vi "Parse Parameters.vi"(6 "error in (no error)":errorcluster, 9 "XML String In":string caption="Entrée de chaîne XML") -> (0 "error out":errorcluster, 3 "Params Values":T1(array[cluster]))   [LabVIEW 2022 SP3, in "EClib functions.lvlib"]
doc: "This intermediate VI transform a cluster of parameters to an array. This transformation is realised by XML Functions."
uses:
  EClib functions.lvlib
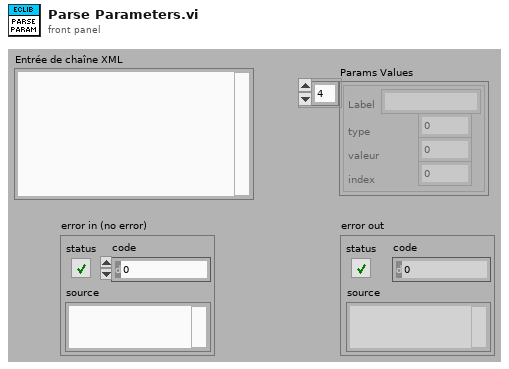
[diagram p1: front panel]
types:
  T1 = cluster{"Label":string, "type":i32, "valeur":u32, "index":i32}[]
  T2 = cluster{"string before end tag":string, i32, i32, i32}[]
  T3 = cluster{"string before end tag":string, i32, u32, i32}
  T4 = cluster{"string before end tag":string, i32, u32, i32}[]
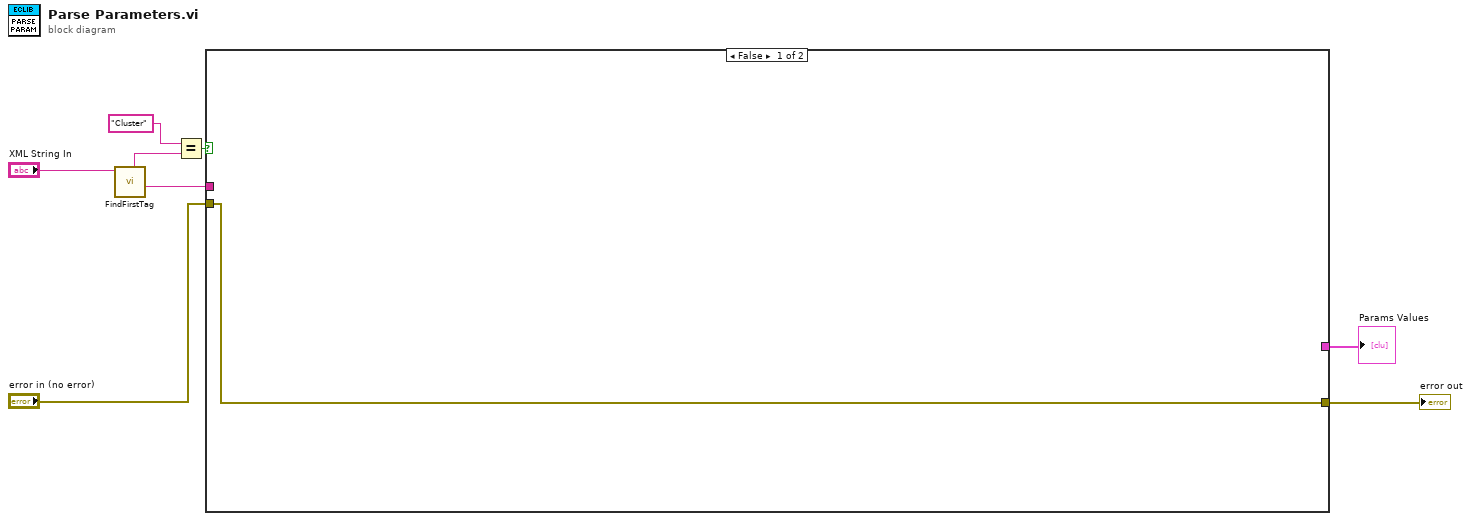
[diagram p0: block diagram]
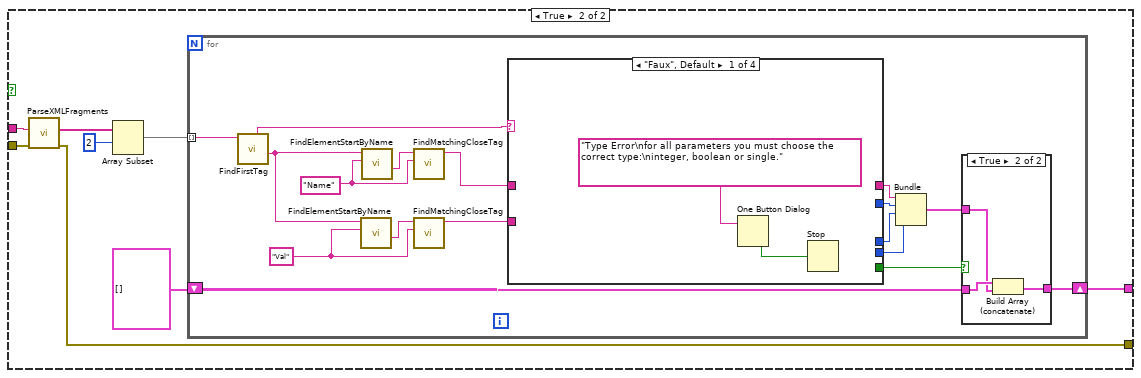
[diagram p2: hidden frame]
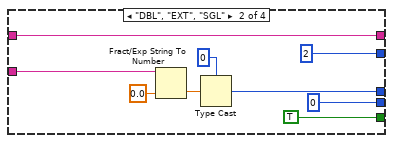
[diagram p4: hidden frame]
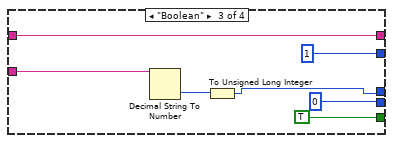
[diagram p5: hidden frame]
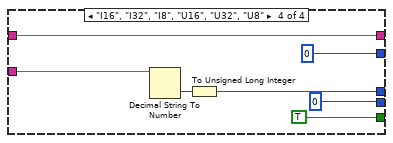
[diagram p6: hidden frame]
diagram:
  n1 = call <vilib>:"FindFirstTag.vi"("XML String In"="XML String In") -> ("after tag"=w7:string, "element name"=w3:string)  [unwired: 5 in, 4 out]
  n2 = Equal?(x="Cluster" ("y"), y=w3) -> (x = y?=w8:bool)
  n3 = case shown="False" w8 {
    tunnel: w7 -> [_ w17]
    tunnel: [_ w12] -> w6
    tunnel: "error in (no error)" -> [w9 w11]
    tunnel: [w9 w10] -> w1
    frame False {
    }
    frame True {
      n4 = call <vilib>:"ParseXMLFragments.vi"("error in (no error)"=w11, "XML in"=w17) -> ("error out"=w10:errorcluster, "XML Elements"=w16:string[])  [unwired: 8 in]
      n5 = Array Subset(array=w16, index=2 ("indice")) -> (w14:string[])  [unwired: 1 in]
      n6 = for {
        tunnel: w14 -> [w34] mode=indexing
        shift-right: [w26] -> w12
        shift-left: T2 [] -> [w28]
        w21 = "Val" ("Element Name")
        w25 = "Name" ("Element Name")
        n7 = call <vilib>:"FindFirstTag.vi"("XML String In"=w34) -> ("after tag"=w33:string, "element name"=w32:string)  [unwired: 5 in, 4 out]
        n8 = call <vilib>:"FindElementStartByName.vi"("Element Name"=w21, "string"=w33) -> ("after substring"=w22:string)  [unwired: 6 in, 3 out]
        n9 = call <vilib>:"FindElementStartByName.vi"("Element Name"=w25, "string"=w33) -> ("after substring"=w24:string)  [unwired: 6 in, 3 out]
        n10 = call <vilib>:"FindMatchingCloseTag.vi"("element name"=w25, "XML string in"=w24) -> ("string before end tag"=w23:string)  [unwired: 5 in, 4 out]
        n11 = call <vilib>:"FindMatchingCloseTag.vi"("element name"=w21, "XML string in"=w22) -> ("string before end tag"=w20:string)  [unwired: 5 in, 4 out]
        n12 = case shown="\"Faux\", Default" w32 {
          tunnel: w20 -> [_ w47 w53 w60]
          tunnel: w23 -> [_ w48 w55 w62]
          tunnel: [_ 2 1 0] -> w31
          tunnel: [_ w48 w55 w62] -> w19
          tunnel: [_ w43 w50 w57] -> w30
          tunnel: [_ TRUE TRUE TRUE] -> w29
          tunnel: [_ 0 0 0] -> w18
          frame "Faux", Default {
            n13 = One Button Dialog(message="Type Error\nfor all parameters you must choose the correct type:\ninteger, boolean or single.") -> (true=w39:bool)  [unwired: 1 in]
            n14 = Stop(stop? (T)=w39) -> ()
          }
          frame "DBL", "EXT", "SGL" {
            n15 = Fract/Exp String To Number(string=w47, default (0 dbl)=sgl 0.0 ("valeur par défaut (0 DBL)")) -> (number=w45:sgl)  [unwired: 2 in, 1 out]
            n16 = Type Cast(type=u32 0, x=w45) -> (*(type *) &x=w43:u32)
          }
          frame "Boolean" {
            n17 = Decimal String To Number(string=w53) -> (number=w51:i32)  [unwired: 2 in, 1 out]
            n18 = To Unsigned Long Integer(number=w51) -> (unsigned 32bit integer=w50:u32)
          }
          frame "I16", "I32", "I8", "U16", "U32", "U8" {
            n19 = Decimal String To Number(string=w60) -> (number=w59:i32)  [unwired: 2 in, 1 out]
            n20 = To Unsigned Long Integer(number=w59) -> (unsigned 32bit integer=w57:u32)
          }
        }
        n21 = Bundle("string before end tag"=w19, w31, w30, w18) -> (w27:T3)  [unwired: 1 in]
        n22 = case shown="True" w29 {
          tunnel: w28 -> [w35 w38]
          tunnel: w27 -> [_ w36]
          tunnel: [w35 w37] -> w26
          frame False {
          }
          frame True {
            n23 = Build Array (concatenate)(w38, w36) -> (w37:T4)
          }
        }
      }
    }
  }
  "Params Values" <- w6
  "error out" <- w1
